vi "Intensity Graph Linecut (Horizontal) (by ref).vi"(6 "Averaging Method":enum16{"Step", "Gaussian"}(ring), 8 "error in (no error)":errorcluster, 9 "width (horizontal)":dbl, 11 "graph_utilities in":refnum<class "graph_utilities.lvclass">) -> (0 "error out":errorcluster, 3 "graph_utilities out":refnum<class "graph_utilities.lvclass">)   [LabVIEW 2019, in "graph_utilities.lvclass"]
doc: "Takes a Horizontal Linecut of an Intensity Graph and outputs to an XY Graph. The center location of the linecut is determined by the y-position of the Intensity Graph curser.\n - <b>width</b> is the standard deviation of a Gaussian function in the units of the Intensity Graph y scale.\n - If <b>width = 0 </b> the spacing between two adjacent data points will be used."
uses:
  graph_utilities.lvclass
  <vilib>/Analysis/baseanly.llb/A x Vector.vi
  <vilib>/Analysis/NI_AALBase.lvlib
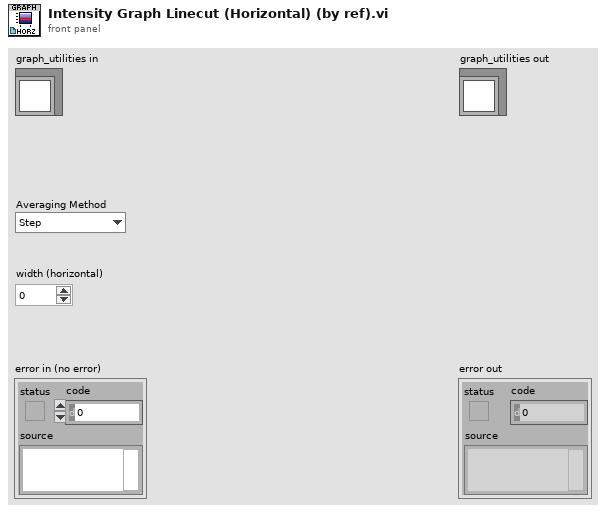
[diagram p1: front panel]
types:
  T1 = typedef "LVPointDoubleTypeDef.ctl" = cluster{"X":dbl, "Y":dbl}
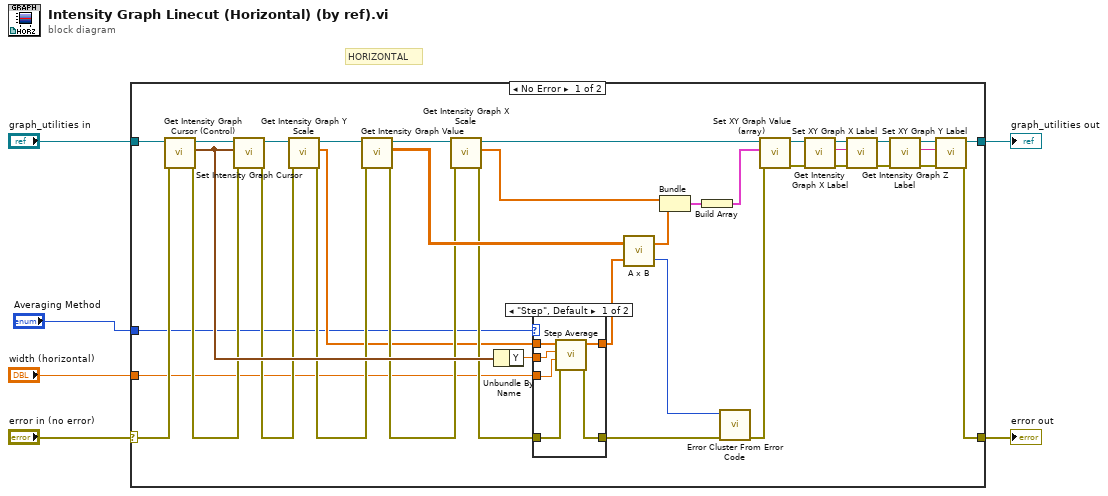
[diagram p0: block diagram]
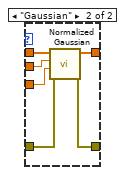
[diagram p2: hidden frame]
diagram:
  # "HORIZONTAL"
  n1 = case shown="No Error" "error in (no error)" {
    selector: "error in (no error)" -> [w33 w58]
    tunnel: [w9 w58] -> w5
    tunnel: [w14 w57] -> w3
    tunnel: "graph_utilities in" -> [w35 w57]
    tunnel: "width (horizontal)" -> [w18 _]
    tunnel: "Averaging Method" -> [w7 _]
    frame No Error {
      n2 = call "Get Intensity Graph Cursor (Control).vi"("error in (no error)"=w33, "graph_utilities in"=w35) -> ("error out"=w32:errorcluster, "Cursor.Cursor Position"=w37:T1, "graph_utilities out"=w36:refnum<class "graph_utilities.lvclass">)  [unwired: 7 in]
      n3 = call "Set Intensity Graph Cursor.vi"("error in (no error)"=w32, "Cursor.Cursor Position"=w37, "graph_utilities in"=w36) -> ("error out"=w31:errorcluster, "graph_utilities out"=w34:refnum<class "graph_utilities.lvclass">)  [unwired: 7 in]
      n4 = call "Get Intensity Graph Y Scale.vi"("error in (no error)"=w31, "graph_utilities in"=w34) -> ("error out"=w30:errorcluster, "Y Scale"=w19:dbl[], "graph_utilities out"=w38:refnum<class "graph_utilities.lvclass">)  [unwired: 6 in, 1 out]
      n5 = call "Get Intensity Graph Value.vi"("error in (no error)"=w30, "graph_utilities in"=w38) -> ("error out"=w29:errorcluster, "Value"=w40:dbl[][], "graph_utilities out"=w39:refnum<class "graph_utilities.lvclass">)  [unwired: 7 in]
      n6 = call "Get Intensity Graph X Scale.vi"("error in (no error)"=w29, "graph_utilities in"=w39) -> ("error out"=w28:errorcluster, "X Scale"=w41:dbl[], "graph_utilities out"=w20:refnum<class "graph_utilities.lvclass">)  [unwired: 6 in, 1 out]
      n7 = Unbundle By Name(w37) -> ("Y"=w43:dbl)
      n8 = case shown="\"Step\", Default" w7 {
        tunnel: [w47 w56] -> w44
        tunnel: w43 -> [w46 w55]
        tunnel: w28 -> [w49 w54]
        tunnel: [w48 w53] -> w27
        tunnel: w19 -> [w50 w52]
        tunnel: w18 -> [w45 w51]
        frame "Step", Default {
          n9 = call "Step Average.vi"("error in (no error)"=w49, "width (c)"=w45, "position (b)"=w46, "Scale"=w50) -> ("error out"=w48:errorcluster, "Averaged Result"=w47:dbl[])  [unwired: 4 in, 2 out]
        }
        frame "Gaussian" {
          n10 = call "Normalized Gaussian.vi"("error in (no error)"=w54, "width (c)"=w51, "position (b)"=w55, "Scale"=w52) -> ("error out"=w53:errorcluster, "Normalized Gaussian"=w56:dbl[])  [unwired: 6 in]
        }
      }
      n11 = call-poly <vilib>:"A x B.vi"("Vector"=w44, "A"=w40) -> ("error"=w42:i32, "A x Vector"=w8:dbl[])
      n12 = Bundle("X Scale"=w41, "A x Vector"=w8) -> (w26:cluster{"X Scale":dbl[], "A x Vector":dbl[]})  [unwired: 1 in]
      n13 = Build Array(w26) -> (w25:cluster{"X Scale":dbl[], "A x Vector":dbl[]}[])
      n14 = call <vilib>:"Error Cluster From Error Code.vi"("error in (no error)"=w27, "error code (0)"=w42) -> ("error out"=w24:errorcluster)  [unwired: 7 in]
      n15 = call "Set XY Graph Value (array).vi"("error in (no error)"=w24, "XY-data"=w25, "graph_utilities in"=w20) -> ("error out"=w10:errorcluster, "graph_utilities out"=w17:refnum<class "graph_utilities.lvclass">)  [unwired: 7 in]
      n16 = call "Get Intensity Graph X Label.vi"("error in (no error)"=w10, "graph_utilities in"=w17) -> ("error out"=w23:errorcluster, "X Label"=w21:string, "graph_utilities out"=w22:refnum<class "graph_utilities.lvclass">)  [unwired: 7 in]
      n17 = call "Set XY Graph X Label.vi"("error in (no error)"=w23, "X Label"=w21, "graph_utilities in"=w22) -> ("error out"=w12:errorcluster, "graph_utilities out"=w13:refnum<class "graph_utilities.lvclass">)  [unwired: 7 in]
      n18 = call "Get Intensity Graph Z Label.vi"("error in (no error)"=w12, "graph_utilities in"=w13) -> ("error out"=w11:errorcluster, "Z Label"=w16:string, "graph_utilities out"=w15:refnum<class "graph_utilities.lvclass">)  [unwired: 7 in]
      n19 = call "Set XY Graph Y Label.vi"("error in (no error)"=w11, "Y Label"=w16, "graph_utilities in"=w15) -> ("error out"=w9:errorcluster, "graph_utilities out"=w14:refnum<class "graph_utilities.lvclass">)  [unwired: 7 in]
    }
    frame Error {
    }
  }
  "error out" <- w5
  "graph_utilities out" <- w3
